vi "Globals.vi"() -> ()   [LabVIEW 2018, in "Stresing_dual_cam.lvclass"]
uses:
  Stresing_dual_cam.lvclass
panel:
  in  "board_sel_offset":u32=3
  in  "cam gain":u32=3
  in  "maddr of IOCTRL":u8=2
  in  "show ADC debug \ninterface":bool=TRUE
  in  "use DAC":bool=TRUE
  in  "maddr of ADC":u8=1
  in  "camera system select":u8=2
  in  "CAMCNT":u32=2
  in  "maddr of CAM":u8
  in  "cam_sel":u8
  in  "nosnobchanged":bool
  in  "board_sel":u32=3
  in  "nob":u32=4
  in  "dioden 2":u16[][](array[numeric])
  in  "dioden 1":u16[][](array[numeric])
  in  "exp time":dbl=0.1
  in  "nos":u32=1100
  in  "PIXEL":u32=1088
  in  "boards":u32=1
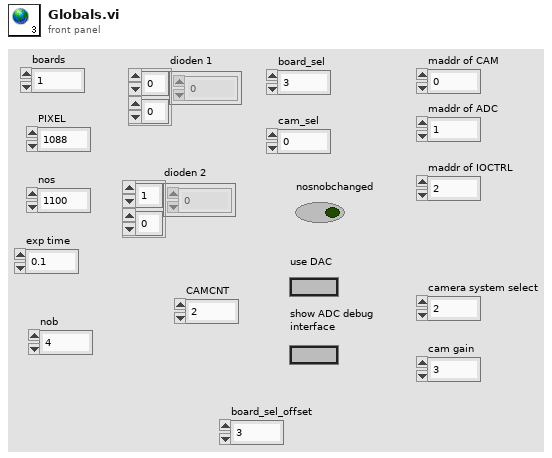
[diagram p1: front panel]
diagram:
